vi "TDMS Write.vi"(7 "Channel Name":string, 8 "error in (no error)":errorcluster, 9 "Group Name":string, 10 "TDMS in":refnum<k34>, 11 "Waveform Array in":refnum<class "Waveform Array.lvclass">) -> (0 "error out":errorcluster, 2 "TDMS Out":refnum<k34>)   [LabVIEW 2020, in "Data.lvlib" / "Waveform Array.lvclass"]
doc: "Write Generic Data to a TDMS file."
uses:
  Waveform Array.lvclass
  Waveform Array.lvclass/Waveform Array.ctl
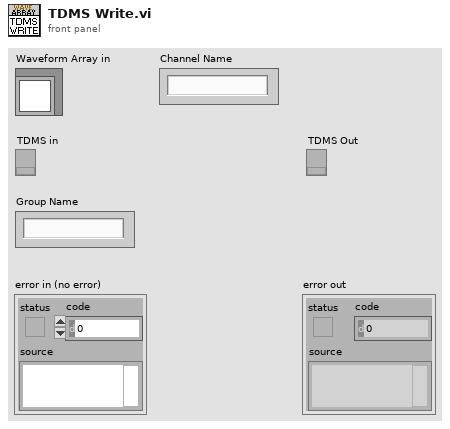
[diagram p1: front panel]
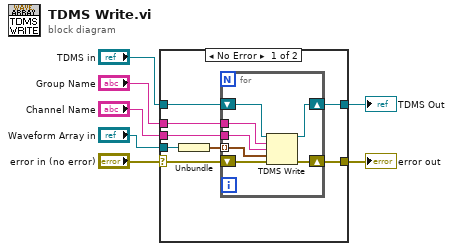
[diagram p0: block diagram]
diagram:
  n1 = case shown="No Error" "error in (no error)" {
    selector: "error in (no error)" -> [w15 w23]
    tunnel: [w14 w23] -> w6
    tunnel: "TDMS in" -> [w13 w24]
    tunnel: [w12 w24] -> w5
    tunnel: "Channel Name" -> [w11 _]
    tunnel: "Group Name" -> [w10 _]
    tunnel: "Waveform Array in" -> [w9 _]
    frame No Error {
      n2 = Unbundle(w9) -> (w8:waveform(dbl)[])
      n3 = for {
        tunnel: w11 -> [w18]
        tunnel: w10 -> [w17]
        tunnel: w8 -> [w16] mode=indexing
        shift-right: [w21] -> w14
        shift-left: w15 -> [w22]
        shift-right: [w19] -> w12
        shift-left: w13 -> [w20]
        n4 = TDMS Write(0:w20, 5:w17, 7:w18, 9:w16, 11:w22) -> (4:w19:refnum<k34>, 15:w21:errorcluster)  [unwired: 1 in, 2 out]
      }
    }
    frame Error {
    }
  }
  "error out" <- w6
  "TDMS Out" <- w5
